vi "ReadWriteSerial.vi"(8 "error in (no error)":errorcluster, 10 "cmd":string, 11 "VISA Refnum in":refnum<visa-resource-name>) -> (0 "error out":errorcluster, 1 "Reply":string, 2 "comm":cluster{"Sent":string, "Received":string}, 3 "VISA Refnum out":refnum<visa-resource-name>)   [LabVIEW 2022 SP3]
uses:
  <vilib>/Utility/error.llb/Trim Whitespace One-Sided.vi
panel:
  out "i":i32
  out "String received":string
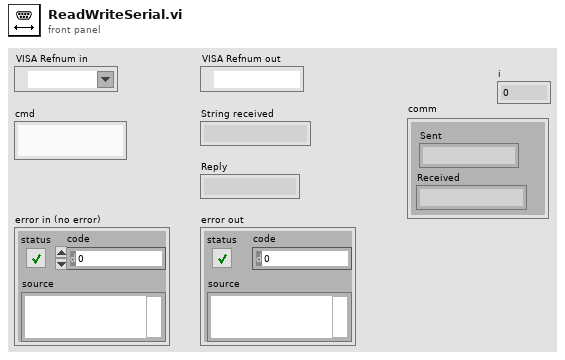
[diagram p1: front panel]
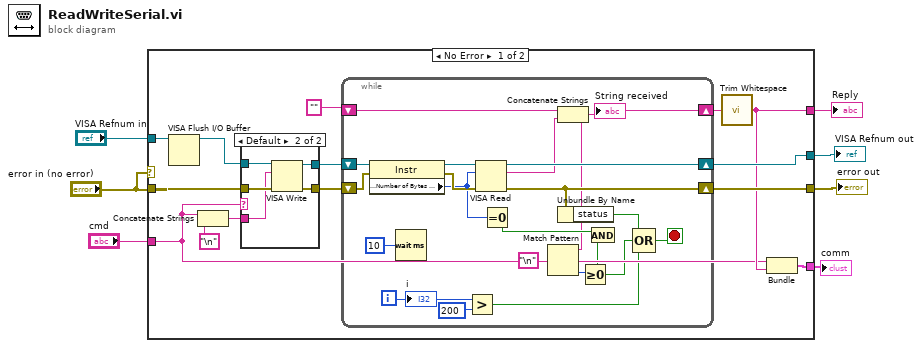
[diagram p0: block diagram]
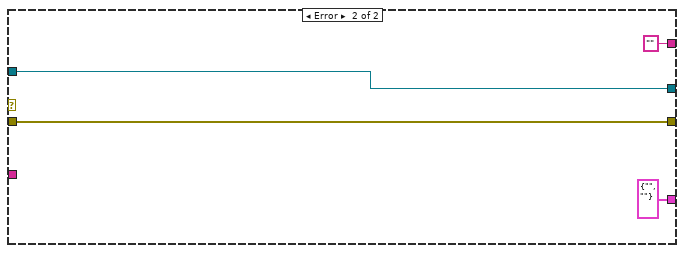
[diagram p3: hidden frame]
diagram:
  n1 = case shown="No Error" "error in (no error)" {
    tunnel: "VISA Refnum in" -> [w18 w49]
    tunnel: "error in (no error)" -> [w17 w50]
    tunnel: [w16 w49] -> w6
    tunnel: [w15 w50] -> w5
    tunnel: [w12 cluster{"cmd":string, "trimmed string":string} {"cmd"="", "trimmed string"=""}] -> w4
    tunnel: [w11 "" ("trimmed string")] -> w3
    tunnel: "cmd" -> [w9 _]
    frame No Error {
      n2 = VISA Flush I/O Buffer(VISA resource name=w18) -> (VISA resource name out=w10:refnum<visa-resource-name>)  [unwired: 2 in, 1 out]
      n3 = Concatenate Strings(w9, "\n" ("regular expression")) -> (w8:string)
      n4 = case shown="Default" w9 {
        tunnel: w17 -> [w22 w28]
        tunnel: w10 -> [w23 w27]
        tunnel: [w23 w26] -> w13
        tunnel: [w22 w25] -> w14
        tunnel: w8 -> [_ w24]
        frame "" {
        }
        frame Default {
          n5 = VISA Write(VISA resource name=w27, write buffer=w24, error in (no error)=w28) -> (VISA resource name out=w26:refnum<visa-resource-name>, error out=w25:errorcluster)  [unwired: 1 out]
        }
      }
      n6 = while {
        shift-right: [w44] -> w16
        shift-left: w13 -> [w46]
        shift-right: [w38] -> w15
        shift-left: w14 -> [w45]
        shift-right: [w33] -> w21
        shift-left: "" -> [w42]
        i -> [w31]
        stop <- w34 stop-if-true
        n7 = property class="Instr"(reference=w46, error in=w45) -> (reference out=w47:refnum<visa-resource-name>, error out=w48:errorcluster, "Serial Settings:Number of Bytes at Serial Port"=w36:u32)
        n8 = Wait (ms)(milliseconds to wait=u32 10) -> ()  [unwired: 1 out]
        n9 = Greater?(x=w31, y=u32 200 ("milliseconds to wait")) -> (0:w29:bool)
        n10 = VISA Read(VISA resource name=w47, byte count=w36, error in (no error)=w48) -> (VISA resource name out=w44:refnum<visa-resource-name>, read buffer=w41:string, error out=w38:errorcluster)  [unwired: 1 out]
        n11 = Equal To 0?(x=w36) -> (x = 0?=w35:bool)
        n12 = Concatenate Strings(w42, w41) -> (w33:string)
        "String received" <- w33
        n13 = Match Pattern(string=w33, regular expression="\n") -> (offset past match=w39:i32)  [unwired: 1 in, 3 out]
        n14 = Unbundle By Name(w38) -> ("status"=w37:bool)
        n15 = Greater Or Equal To 0?(x=w39) -> (x >= 0?=w32:bool)
        n16 = And(x=w35, y=w32) -> ()  [unwired: 1 out]
        n17 = Compound Arithmetic op=OR(w37, w32, w29) -> (w34:bool)
        "i" <- w31
      }
      n18 = call <vilib>:"Trim Whitespace.vi"("string"=w21) -> ("trimmed string"=w11:string)  [unwired: 1 in]
      n19 = Bundle("cmd"=w9, "trimmed string"=w11) -> (w12:cluster{"cmd":string, "trimmed string":string})  [unwired: 1 in]
    }
    frame Error {
    }
  }
  "VISA Refnum out" <- w6
  "error out" <- w5
  "comm" <- w4
  "Reply" <- w3
